vi "Do.vi"(8 "error in (no error)":errorcluster, 10 "Actor in":refnum<class "Actor.lvclass">, 11 "NotificationMessageAdapter":refnum<class "NotificationMessageAdapter.lvclass">) -> (0 "error out":errorcluster, 2 "Actor out":refnum<class "Actor.lvclass">)   [LabVIEW 2017, in "ActorMessageTransport.lvlib" / "NotificationMessageAdapter.lvclass"]
doc: "(<B>Filename</B>: Actor Framework.lvlib:Message.lvclass:Do.vi)\n\nDefines what a message does when it is received by an actor. Generally, a message instructs an actor to invoke one of its methods. By default, this method does nothing. A child class must override it to define behavior."
uses:
  NotificationMessageAdapter.lvclass
  <vilib>/ActorFramework/Actor/Actor.lvclass
  NotificationMessageAdapter.lvclass/NotificationMessageAdapter.ctl
  <vilib>/ActorFramework/Message/Message.lvclass
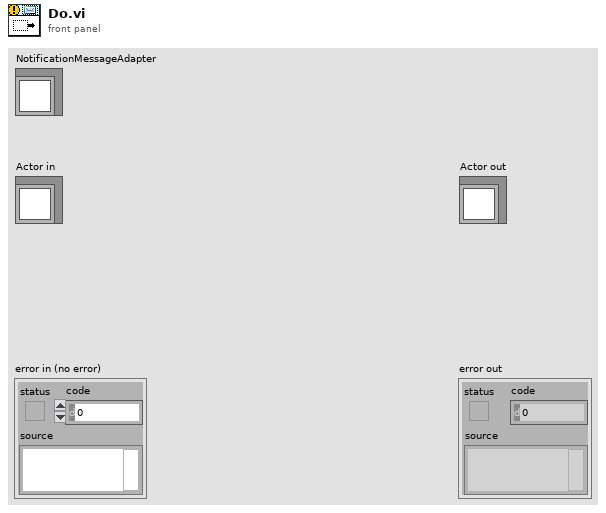
[diagram p1: front panel]
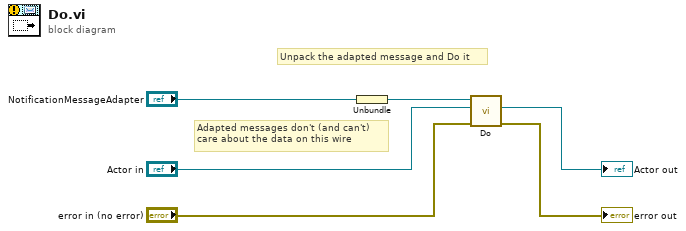
[diagram p0: block diagram]
diagram:
  # "Adapted messages don't (and can't)\ncare about the data on this wire"
  # "Unpack the adapted message and Do it"
  n1 = Unbundle("NotificationMessageAdapter") -> (w1:refnum<class "Message.lvclass">)
  n2 = call-dynamic "Do.vi"("error in (no error)"="error in (no error)", "Actor in"="Actor in", "Message"=w1) -> ("error out"=→"error out":errorcluster, "Actor out"=→"Actor out":refnum<class "Actor.lvclass">)  [unwired: 7 in]
